vi "Connect.vi"(8 "error in":errorcluster, 11 "57XX in":refnum<class "57XX.lvclass">) -> (0 "error out":errorcluster, 3 "57XX out":refnum<class "57XX.lvclass">)   [LabVIEW 2019, in "57XX.lvlib" / "57XX.lvclass"]
uses:
  Library/57XX.lvclass
  C:/Users/Public/Documents/Development/builds/Instruments/Instruments.lvlibp/Library/Instruments.lvclass
  Library/57XX.lvclass/57XX.ctl
  builds/Instruments/Instruments.lvlibp/Accessors/Read Resource.vi
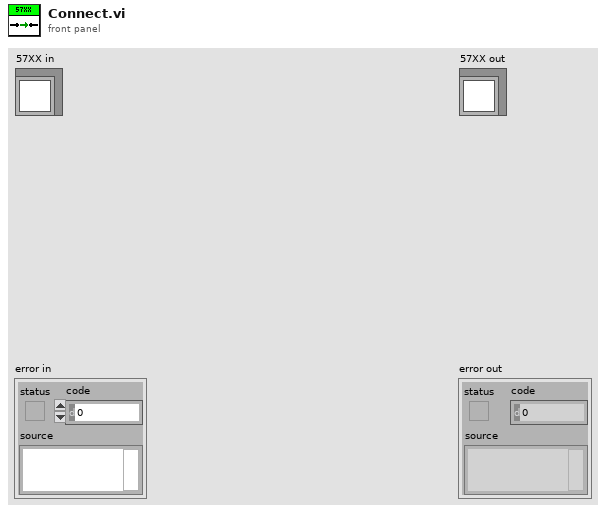
[diagram p1: front panel]
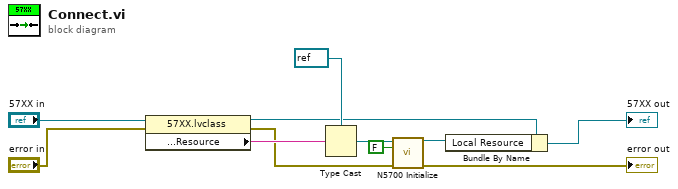
[diagram p0: block diagram]
diagram:
  n1 = property class="57XX.lvclass"(reference="57XX in", error in="error in") -> (reference out=w6:refnum<class "57XX.lvclass">, error out=w4:errorcluster, "Accessors:Configuration:Resource"=w11:string)
  n2 = Type Cast(type=refnum<visa-resource-name> refnum ("VISA name"), x=w11) -> (*(type *) &x=w9:refnum<visa-resource-name>)
  n3 = call <instrlib>:"N5700 Initialize.vi"("VISA name"=w9, "ID Query (T)"=FALSE, "error in (no error)"=w4) -> ("VISA out"=w7:refnum<visa-resource-name>, "error out"=→"error out":errorcluster)  [unwired: 11 in]
  n4 = Bundle By Name(cluster=w6, "Local Resource"=w7) -> (→"57XX out":refnum<class "57XX.lvclass">)
